vi "lecor.vi"(3 "Parâmetros 2":T2={"Azul Max EV3 Cor"=17, "Azul Min EV3 Cor"=0, "Verde Max EV3 Cor"=6, "Verde Min EV3 Cor"=0, "Vermelho Max Ev3 Cor"=0, "Vermelho Min EV3 Cor"=0, "Chão EV3 Cor"=0.0, "Branco Max EV3 Cor"=0.0, "Branco Min EV3 Cor"=0.0, "Preto Max EV3 Cor"=0.0, "Preto Min EV3 Cor"=0.0, "Distância Tubulação"=0.0, "Distância Frontal"=0.0, "Amarelo Max EV3 Cor"=0.0, "Amarelo Min EV3 Cor"=0.0, "Distância Lateral"=0.0, "90°"=0.0, "180°"=0.0, "Seguidor de Linha"=0.0}, 5 "NXT/EV3":T1) -> (0 "cor":dbl, 2 "NXT/EV3 2":T1)   [LabVIEW 2016]
uses:
  <vilib>/NXT/Subs/LVHSConnector.ctl
  <vilib>/NXT/LegoClasses/BrickReference/BrickReference.lvclass
  <vilib>/NXT/Block Support/NXT_InputPort.ctl
  <vilib>/NXT/Dual Mode Library/Sensors/EV3_Color_Reflect.vi
  <vilib>/NXT/NXTIO Xnodes/AddressXNode/NXTIOAddress.xnode
panel:
  # "Sensor EV3 Cor"
  # "Sensor Ultrassônico"
  # "Sensor Giroscópio"
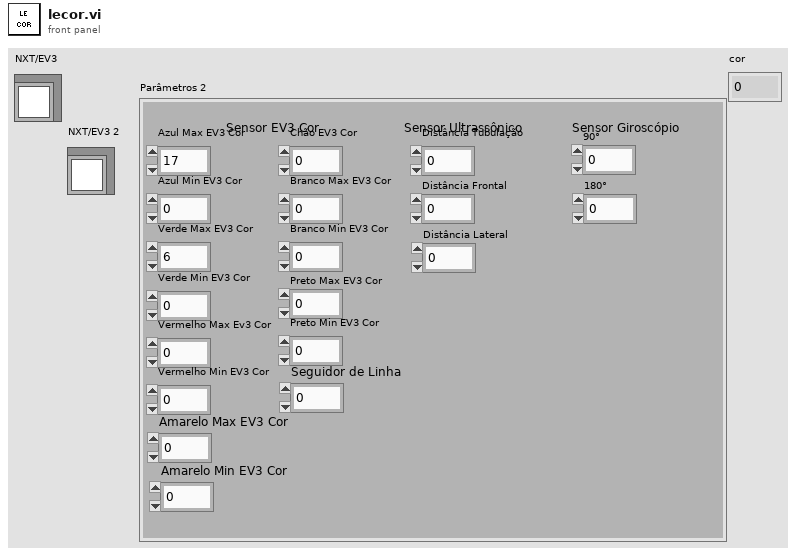
[diagram p1: front panel]
types:
  T1 = typedef "LVHSConnector.ctl" = refnum<class "BrickReference.lvclass">
  T2 = cluster{"Azul Max EV3 Cor":i32, "Azul Min EV3 Cor":i32, "Verde Max EV3 Cor":i32, "Verde Min EV3 Cor":i32, "Vermelho Max Ev3 Cor":i32, "Vermelho Min EV3 Cor":i32, "Chão EV3 Cor":sgl, "Branco Max EV3 Cor":sgl, "Branco Min EV3 Cor":sgl, "Preto Max EV3 Cor":sgl, "Preto Min EV3 Cor":sgl, "Distância Tubulação":sgl, "Distância Frontal":sgl, "Amarelo Max EV3 Cor":dbl, "Amarelo Min EV3 Cor":dbl, "Distância Lateral":sgl, "90°":sgl, "180°":sgl, "Seguidor de Linha":dbl}
  T3 = typedef "NXT_InputPort.ctl" = u32
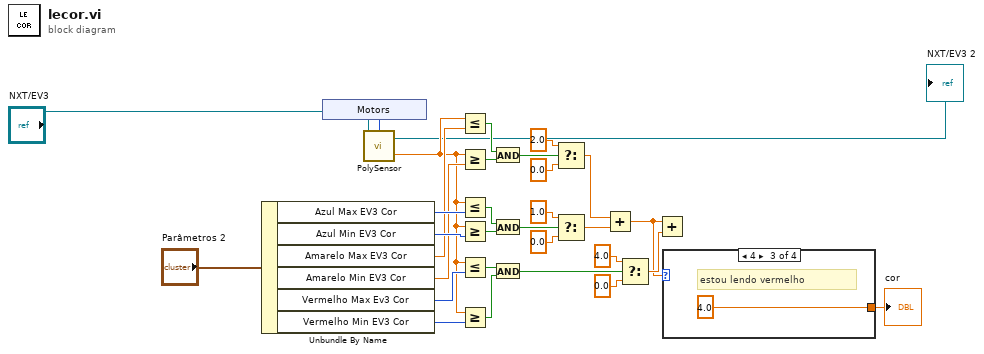
[diagram p0: block diagram]
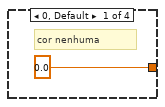
[diagram p2: hidden frame]
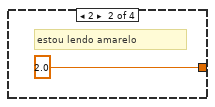
[diagram p3: hidden frame]
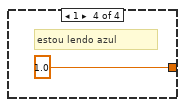
[diagram p4: hidden frame]
diagram:
  n1 = Unbundle By Name("Parâmetros 2") -> ("Azul Max EV3 Cor"=w27:i32, "Azul Min EV3 Cor"=w26:i32, "Amarelo Max EV3 Cor"=w20:dbl, "Amarelo Min EV3 Cor"=w19:dbl, "Vermelho Max Ev3 Cor"=w11:i32, "Vermelho Min EV3 Cor"=w10:i32)
  n2 = xnode "Motors"() -> ("Sensor"=w31:T3)
  n3 = call-poly <vilib>:"PolySensor.vi"("NXT/EV3"="NXT/EV3", "Port (Port 1)"=w31) -> ("Scaled Value"=w9:sgl, "NXT/EV3"=→"NXT/EV3 2":T1)  [unwired: 1 in]
  n4 = Less Or Equal?(x=w9, y=w20) -> (x <= y?=w18:bool)
  n5 = Greater Or Equal?(x=w9, y=w19) -> (x >= y?=w17:bool)
  n6 = Less Or Equal?(x=w9, y=w27) -> (x <= y?=w28:bool)
  n7 = Greater Or Equal?(x=w9, y=w26) -> (x >= y?=w29:bool)
  n8 = Less Or Equal?(x=w9, y=w11) -> (x <= y?=w13:bool)
  n9 = Greater Or Equal?(x=w9, y=w10) -> (x >= y?=w14:bool)
  n10 = And(x=w18, y=w17) -> (x .and. y?=w16:bool)
  n11 = And(x=w28, y=w29) -> (x .and. y?=w25:bool)
  n12 = And(x=w13, y=w14) -> (x .and. y?=w15:bool)
  n13 = Select(t=2.0, s=w16, f=0.0) -> (s? t:f=w6:dbl)
  n14 = Select(t=1.0, s=w25, f=0.0) -> (s? t:f=w7:dbl)
  n15 = Add(x=w6, y=w7) -> (x+y=w4:dbl)
  n16 = Select(t=4.0, s=w15, f=0.0) -> (s? t:f=w5:dbl)
  n17 = Add(x=w4, y=w5) -> ()  [unwired: 1 out]
  n18 = case shown="4" w4 {
    tunnel: [0.0 ("t") 2.0 ("t") 4.0 ("t") 1.0 ("t")] -> w1
    frame 0, Default {
      # "cor nenhuma"
    }
    frame 2 {
      # "estou lendo amarelo"
    }
    frame 4 {
      # "estou lendo vermelho"
    }
    frame 1 {
      # "estou lendo azul"
    }
  }
  "cor" <- w1
